vi "issueInfo.get.vi"(11 "issue_class in":refnum<class "issue_class.lvclass">) -> (2 "issueInfo":T1, 3 "issue_class out":refnum<class "issue_class.lvclass">)   [LabVIEW 2024, in "issue_class.lvclass"]
uses:
  issue_class.lvclass
  comic_class/issueInfo--cluster.ctl
  comic_class/creator--cluster.ctl
  comic_class/character--cluster.ctl
  comic_class/team--cluster.ctl
  comic_class/location--cluster.ctl
  comic_class/concept--cluster.ctl
  comic_class/thing--cluster.ctl
  comic_class/storyArc--cluster.ctl
  issue_class.lvclass/issue_class.ctl
  comic_class/comic_class.lvclass
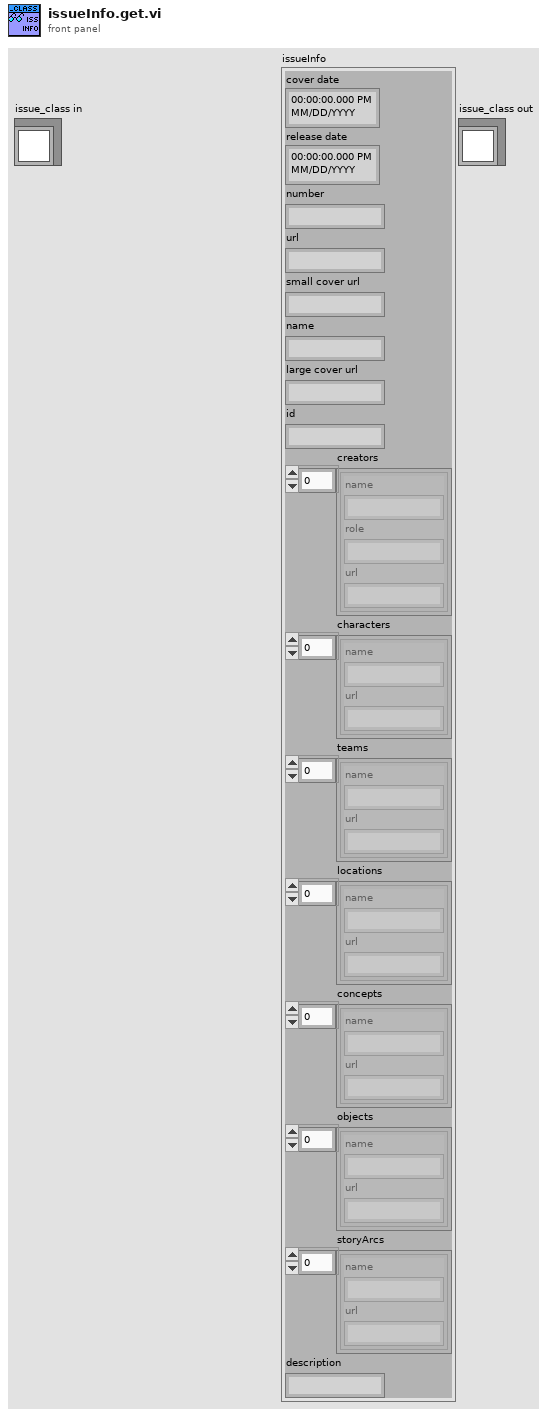
[diagram p1: front panel]
types:
  T1 = typedef "comic_class.lvclass/issueInfo--cluster.ctl" = cluster{"cover date":timestamp, "release date":timestamp, "number":string, "url":string, "small cover url":string, "name":string, "large cover url":string, "id":string, "creators":T2[], "characters":T3[], "teams":T4[], "locations":T5[], "concepts":T6[], "objects":T7[], "storyArcs":T8[], "description":string}
  T2 = typedef "comic_class.lvclass/creator--cluster.ctl" = cluster{"name":string, "role":string, "url":string}
  T3 = typedef "comic_class.lvclass/character--cluster.ctl" = cluster{"name":string, "url":string}
  T4 = typedef "comic_class.lvclass/team--cluster.ctl" = cluster{"name":string, "url":string}
  T5 = typedef "comic_class.lvclass/location--cluster.ctl" = cluster{"name":string, "url":string}
  T6 = typedef "comic_class.lvclass/concept--cluster.ctl" = cluster{"name":string, "url":string}
  T7 = typedef "comic_class.lvclass/thing--cluster.ctl" = cluster{"name":string, "url":string}
  T8 = typedef "comic_class.lvclass/storyArc--cluster.ctl" = cluster{"name":string, "url":string}
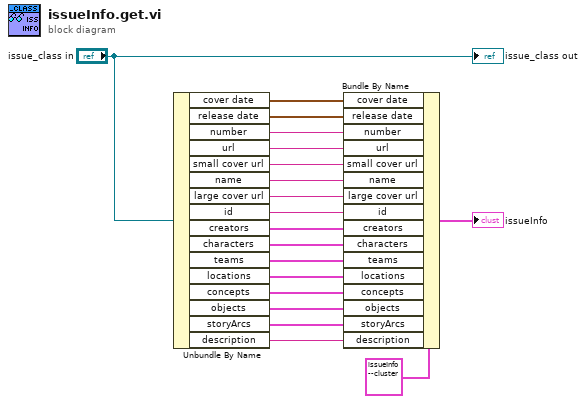
[diagram p0: block diagram]
diagram:
  n1 = Unbundle By Name("issue_class in") -> ("cover date"=w18:timestamp, "release date"=w17:timestamp, "number"=w16:string, "url"=w15:string, "small cover url"=w14:string, "name"=w13:string, "large cover url"=w12:string, "id"=w11:string, "creators"=w10:T2[], "characters"=w9:T3[], "teams"=w8:T4[], "locations"=w7:T5[], "concepts"=w6:T6[], "objects"=w5:T7[], "storyArcs"=w4:T8[], "description"=w1:string)
  n2 = Bundle By Name(cluster=T1 {"cover date"=timestamp(0 s since 1904-01-01), "release date"=timestamp(0 s since 1904-01-01), "number"="", "url"="", "small cover url"="", "name"="", "large cover url"="", "id"="", "creators"=[], "characters"=[], "teams"=[], "locations"=[], "concepts"=[], "objects"=[], "storyArcs"=[], "description"=""} ("issueInfo"), "cover date"=w18, "release date"=w17, "number"=w16, "url"=w15, "small cover url"=w14, "name"=w13, "large cover url"=w12, "id"=w11, "creators"=w10, "characters"=w9, "teams"=w8, "locations"=w7, "concepts"=w6, "objects"=w5, "storyArcs"=w4, "description"=w1) -> (→"issueInfo":T1)
  "issue_class out" <- "issue_class in"
